vi "Experiment04.vi"() -> ()   [LabVIEW 2009]
uses:
  <vilib>/imath/engines/lvmath2/RunTimeEngine/ErrorHandling/NIMS_Finalize Error.vi
  <vilib>/imath/engines/lvmath2/RunTimeEngine/Parser/MC_Version.vi
  <vilib>/imath/engines/lvmath2/RunTimeEngine/Managers/WorkSpace/UID Generator.vi
  <vilib>/imath/engines/lvmath2/RunTimeEngine/NodeEndStatement/NIMS_NodeEndStatement_Output.vi
  <instcachedir>/0/NIMS_NodeEndStatement_Output_B70DDD75627E4997AAE11E9955EDAA25.lvgen/NIMS_NodeEndStatement_Output_B70DDD75627E4997AAE11E9955EDAA25_000.vi
  <vilib>/imath/engines/lvmath2/RunTimeEngine/Managers/SymbolTable/Clear UID.vi
  <vilib>/imath/engines/lvmath2/RunTimeEngine/LocalVariableDefStatement/MC_LocalVariableDefStatement_Display.vi
  <vilib>/imath/engines/lvmath2/RunTimeEngine/RunTimeType/NIMS_RunTimeType_From StrictType (excl LVString).vi
  <vilib>/imath/engines/lvmath2/RunTimeEngine/RangeToken/NIMS_Range.vi
  <instcachedir>/0/NIMS_Range_6D647EC16A744C98B5DE1D649A2D648D.lvgen/NIMS_Range_6D647EC16A744C98B5DE1D649A2D648D_001.vi
  <vilib>/imath/engines/lvmath/Functions/Error Handling/error.ctl
  <vilib>/imath/engines/lvmath/Functions/Error Handling/MergeErrorsWrapper.vi
  <vilib>/imath/engines/lvmath2/RunTimeEngine/VariableToken/NIMS_VariableToken_CondDefined.vi
  <instcachedir>/0/NIMS_VariableToken_CondDefined_5641E79000FB4D628475532441475385.lvgen/NIMS_VariableToken_CondDefined_5641E79000FB4D628475532441475385_001.vi
  <vilib>/imath/engines/lvmath/Functions/Error Handling/MC_Mask_Errors.vi
  <vilib>/imath/engines/lvmath2/RunTimeEngine/BuiltInFunctions/rem/NIMS_rem_no checks.vi
  <instcachedir>/0/NIMS_rem_no checks_4CC9B305AB7E42EF90AFC4973FB32F8D.lvgen/NIMS_rem_no checks_4CC9B305AB7E42EF90AFC4973FB32F8D_000.vi
  <vilib>/imath/engines/lvmath2/RunTimeEngine/BuiltInFunctions/uint32/NIMS_uint32(real).vi
  <instcachedir>/0/NIMS_uint32(real)_FDC83D68D45943DDB8F3F934FF8A712F.lvgen/NIMS_uint32(real)_FDC83D68D45943DDB8F3F934FF8A712F_000.vi
  <vilib>/imath/engines/lvmath2/RunTimeEngine/BuiltInFunctions/double/NIMS_double.vi
  <instcachedir>/0/NIMS_double_2CE444F3CE4146B199A482FE12545E45.lvgen/NIMS_double_2CE444F3CE4146B199A482FE12545E45_000.vi
  <vilib>/imath/engines/lvmath2/RunTimeEngine/BuiltInFunctions/length/NIMS_length(GV).vi
  <instcachedir>/0/NIMS_length(GV)_7D6E94E728E145E68721C53861296D96.lvgen/NIMS_length(GV)_7D6E94E728E145E68721C53861296D96_000.vi
  <instcachedir>/0/NIMS_Range_6D647EC16A744C98B5DE1D649A2D648D.lvgen/NIMS_Range_6D647EC16A744C98B5DE1D649A2D648D_000.vi
  <vilib>/imathl/engines/lvmath/Functions/Error Handling/Create Error.vi
  <vilib>/imath/engines/lvmath2/RunTimeEngine/ReplaceToken/NIMS_Replace - V(S)=S.vi
  <instcachedir>/0/NIMS_Replace - V(S)=S_670A9E0533664C1D848C8E58B3321B6A.lvgen/NIMS_Replace - V(S)=S_670A9E0533664C1D848C8E58B3321B6A_002.vi
  <vilib>/imath/engines/lvmath2/RunTimeEngine/ReplaceToken/NIMS_Replace - Size Check _(_)=S.vi
  <instcachedir>/0/NIMS_Replace - Size Check _(_)=S_8596181D73404097BAB9CBB006194BB0.lvgen/NIMS_Replace - Size Check _(_)=S_8596181D73404097BAB9CBB006194BB0_002.vi
  <vilib>/imath/engines/lvmath2/RunTimeEngine/ReplaceToken/NIMS_Replace - Check Linear.vi
  <instcachedir>/0/NIMS_Replace - Check Linear_9243CBB174894FF6977027453DA6955E.lvgen/NIMS_Replace - Check Linear_9243CBB174894FF6977027453DA6955E_002.vi
  <vilib>/imath/engines/lvmath2/RunTimeEngine/VariableToken/NIMS_VariableToken_CondDefinedDefinedByReplace.vi
  <instcachedir>/0/NIMS_VariableToken_CondDefinedDefinedByReplace_D162CFFC24174562A9FEA619A91E1A56.lvgen/NIMS_VariableToken_CondDefinedDefinedByReplace_D162CFFC24174562A9FEA619A91E1A56_002.vi
  <vilib>/imath/engines/lvmath2/RunTimeEngine/CommandStatement/MC_CommandStatement_break.vi
  <vilib>/imath/engines/lvmath2/RunTimeEngine/ArithmeticOperatorToken/NIMS_ArithmeticOperator_times.vi
  <instcachedir>/0/NIMS_ArithmeticOperator_times_3987BC660D7947CD8628C10658A43225.lvgen/NIMS_ArithmeticOperator_times_3987BC660D7947CD8628C10658A43225_001.vi
  <instcachedir>/0/NIMS_NodeEndStatement_Output_B70DDD75627E4997AAE11E9955EDAA25.lvgen/NIMS_NodeEndStatement_Output_B70DDD75627E4997AAE11E9955EDAA25_001.vi
  <instcachedir>/0/NIMS_ArithmeticOperator_times_3987BC660D7947CD8628C10658A43225.lvgen/NIMS_ArithmeticOperator_times_3987BC660D7947CD8628C10658A43225_000.vi
  <vilib>/imath/engines/lvmath2/RunTimeEngine/VariableToken/Read/NIMS_Get Elements - RV(_) - Check.vi
  <instcachedir>/0/NIMS_Get Elements - RV(_) - Check_60F12861D0564803969A5D0D0D1716CD.lvgen/NIMS_Get Elements - RV(_) - Check_60F12861D0564803969A5D0D0D1716CD_000.vi
  <instcachedir>/0/NIMS_VariableToken_CondDefined_5641E79000FB4D628475532441475385.lvgen/NIMS_VariableToken_CondDefined_5641E79000FB4D628475532441475385_000.vi
  <instcachedir>/0/NIMS_VariableToken_CondDefined_5641E79000FB4D628475532441475385.lvgen/NIMS_VariableToken_CondDefined_5641E79000FB4D628475532441475385_003.vi
  <vilib>/imath/engines/lvmath2/RunTimeEngine/ArithmeticOperatorToken/NIMS_ArithmeticOperator_power(S).vi
  <instcachedir>/0/NIMS_ArithmeticOperator_power(S)_A502679C095F4520BDC53E297C98A9BD.lvgen/NIMS_ArithmeticOperator_power(S)_A502679C095F4520BDC53E297C98A9BD_000.vi
  <vilib>/imath/engines/lvmath2/RunTimeEngine/BuiltInFunctions/abs/NIMS_abs(signed).vi
  <instcachedir>/0/NIMS_abs(signed)_C4FCB8E6058B49B797C7C8D53CA5F6EC.lvgen/NIMS_abs(signed)_C4FCB8E6058B49B797C7C8D53CA5F6EC_000.vi
  <instcachedir>/0/NIMS_Replace - V(S)=S_670A9E0533664C1D848C8E58B3321B6A.lvgen/NIMS_Replace - V(S)=S_670A9E0533664C1D848C8E58B3321B6A_001.vi
  <instcachedir>/0/NIMS_Replace - Size Check _(_)=S_8596181D73404097BAB9CBB006194BB0.lvgen/NIMS_Replace - Size Check _(_)=S_8596181D73404097BAB9CBB006194BB0_001.vi
  <instcachedir>/0/NIMS_Replace - Check Linear_9243CBB174894FF6977027453DA6955E.lvgen/NIMS_Replace - Check Linear_9243CBB174894FF6977027453DA6955E_001.vi
  <instcachedir>/0/NIMS_VariableToken_CondDefinedDefinedByReplace_D162CFFC24174562A9FEA619A91E1A56.lvgen/NIMS_VariableToken_CondDefinedDefinedByReplace_D162CFFC24174562A9FEA619A91E1A56_001.vi
  <instcachedir>/0/NIMS_Replace - V(S)=S_670A9E0533664C1D848C8E58B3321B6A.lvgen/NIMS_Replace - V(S)=S_670A9E0533664C1D848C8E58B3321B6A_000.vi
  <instcachedir>/0/NIMS_Replace - Size Check _(_)=S_8596181D73404097BAB9CBB006194BB0.lvgen/NIMS_Replace - Size Check _(_)=S_8596181D73404097BAB9CBB006194BB0_000.vi
  <instcachedir>/0/NIMS_Replace - Check Linear_9243CBB174894FF6977027453DA6955E.lvgen/NIMS_Replace - Check Linear_9243CBB174894FF6977027453DA6955E_000.vi
  <instcachedir>/0/NIMS_VariableToken_CondDefinedDefinedByReplace_D162CFFC24174562A9FEA619A91E1A56.lvgen/NIMS_VariableToken_CondDefinedDefinedByReplace_D162CFFC24174562A9FEA619A91E1A56_000.vi
  <instcachedir>/0/NIMS_abs(signed)_C4FCB8E6058B49B797C7C8D53CA5F6EC.lvgen/NIMS_abs(signed)_C4FCB8E6058B49B797C7C8D53CA5F6EC_001.vi
  <instcachedir>/0/NIMS_NodeEndStatement_Output_B70DDD75627E4997AAE11E9955EDAA25.lvgen/NIMS_NodeEndStatement_Output_B70DDD75627E4997AAE11E9955EDAA25_002.vi
  <vilib>/imath/engines/lvmath2/RunTimeEngine/Managers/SymbolTable/NIMS_WorkSpace.lvlib
panel:
  out "Current VI path 10":string
  out "New Path for Picture 10":string
  out "Part Stripped 10":string
  out "Stripped Path 10":string
  out "Current VI path 9":string
  out "New Path for Picture 9":string
  out "Part Stripped 9":string
  out "Stripped Path 9":string
  out "Current VI path 8":string
  out "New Path for Picture 8":string
  out "Part Stripped 8":string
  out "Stripped Path 8":string
  out "Current VI path 7":string
  out "New Path for Picture 7":string
  out "Part Stripped 7":string
  out "Stripped Path 7":string
  out "Current VI path 6":string
  out "New Path for Picture 6":string
  out "Part Stripped 6":string
  out "Stripped Path 6":string
  out "Current VI path 5":string
  out "New Path for Picture 5":string
  out "Part Stripped 5":string
  out "Stripped Path 5":string
  out "Current VI path 4":string
  out "New Path for Picture 4":string
  out "Part Stripped 4":string
  out "Stripped Path 4":string
  out "Current VI path 3":string
  out "New Path for Picture 3":string
  out "Part Stripped 3":string
  out "Stripped Path 3":string
  out "Current VI path 2":string
  out "New Path for Picture 2":string
  out "Part Stripped 2":string
  out "Stripped Path 2":string
  out "Current VI path":string
  out "New Path for Picture":string
  out "Part Stripped":string
  out "Stripped Path":string
  out "error out":errorcluster
  out "error out":errorcluster
  out "error out":errorcluster
  out "error out":errorcluster
  in  "?":enum32{"CAVITY"}(tab)
  in  "FIRST 3dB POINT":bool
  in  "?":dbl(slide) scale=8.0..12.5 scale format="%#.6g"
  out "Qdesigned":dbl
  in  "RESONANT FREQUENCY":dbl(slide) scale=8.5..12.0
  out "?":errorcluster
  out "XY Graph":cluster{"Y":dbl[], "Y":dbl[]}[](graph)
  out "frequency":dbl
  out "power(dB)":cdb
  in  "SECOND 3dB POINT":bool
  in  "BAND WIDTH":bool
  in  "Q FACTOR":bool
  in  "POWER(dB) at RESONANCE":bool
  out "?":dbl
  out "?":dbl
  out "?":dbl
  out "?":dbl
  out "?":dbl
  in  "HELP FOR CAVITY":bool
  in  "?":enum32{"ATTENUATOR"}(tab)
  out "?":dbl[](graph)
  in  "Set the value of attenuation in dB":dbl(slide) scale=0.0..100.0
  out "?":errorcluster
  in  "HELP FOR ATTENUATOR":bool
  out "error out":errorcluster
  in  "?":enum32{"ISOLATOR"}(tab)
  out "?":dbl[](graph)
  in  "?":bool
  out "?":errorcluster
  in  "HELP FOR ISOLATOR":bool
  in  "?":enum32{"MODULATOR"}(tab)
  out "?":dbl[](graph)
  in  "Modulating Frequency(KHz)":dbl(slide) scale=0.5..1.5
  out "?":errorcluster
  in  "HELP FOR MODULATOR":bool
  in  "?":enum32{"SOURCE"}(tab)
  out "?":dbl[](graph)
  in  "Frequency of carrier wave(GHz)":dbl(slide) scale=8.2..12.4
  in  "Voltage 3":dbl(knob) scale=0.0..20.0 scale format="%#_10g"
  out "?":errorcluster
  in  "HELP FOR SOURCE":bool
  # "Backward Direction"
  # "Forward direction"
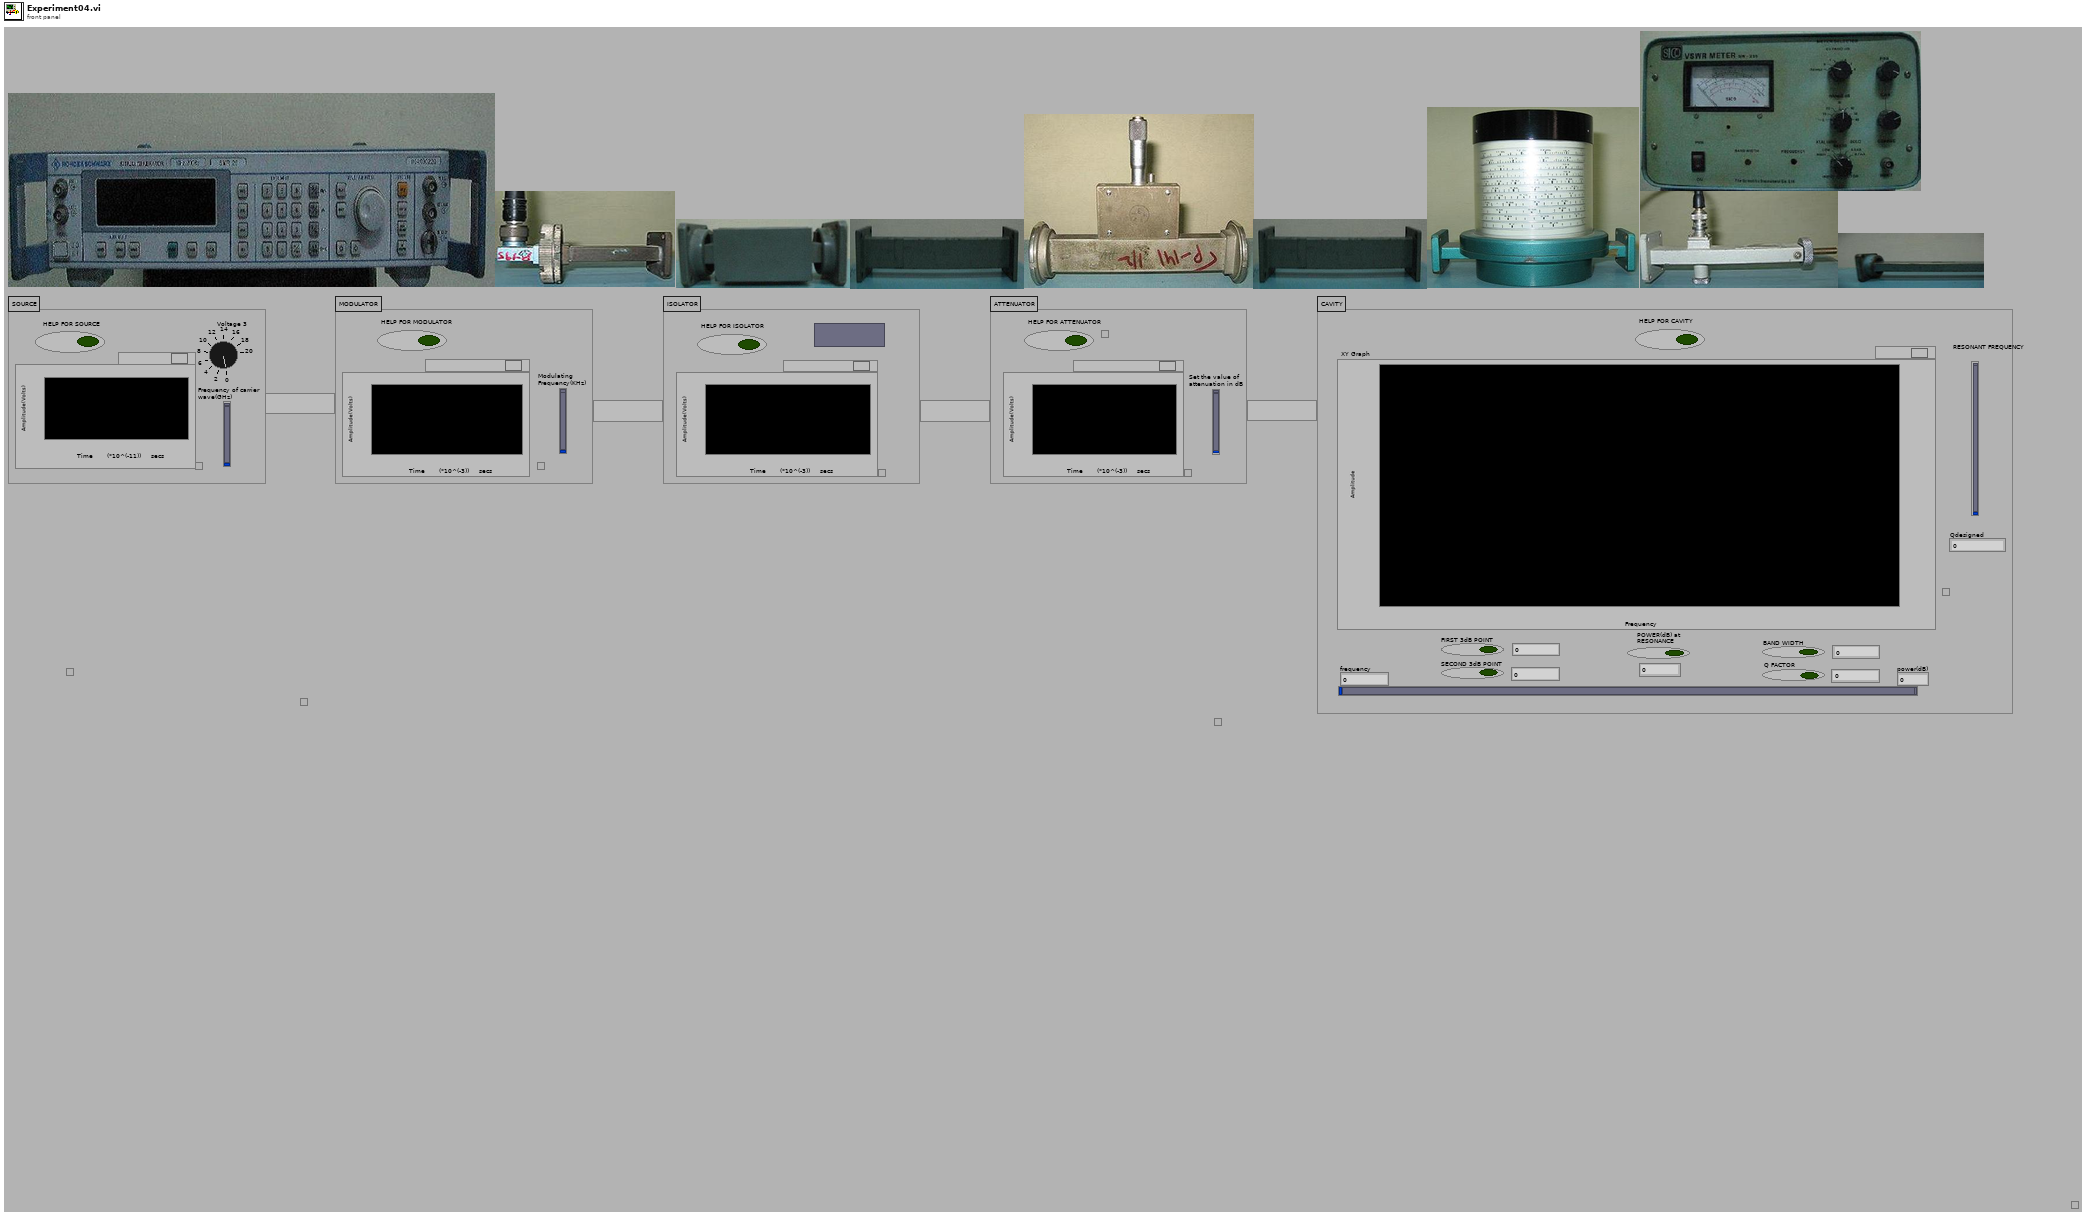
[diagram p1: front panel]
types:
  T1 = typedef "imagedata.ctl" = cluster{"image type":i32, "image depth":i32, "image":u8[], "mask":u8[], "colors":u32[], "Rectangle":cluster{"left":i16, "top":i16, "right":i16, "bottom":i16}}
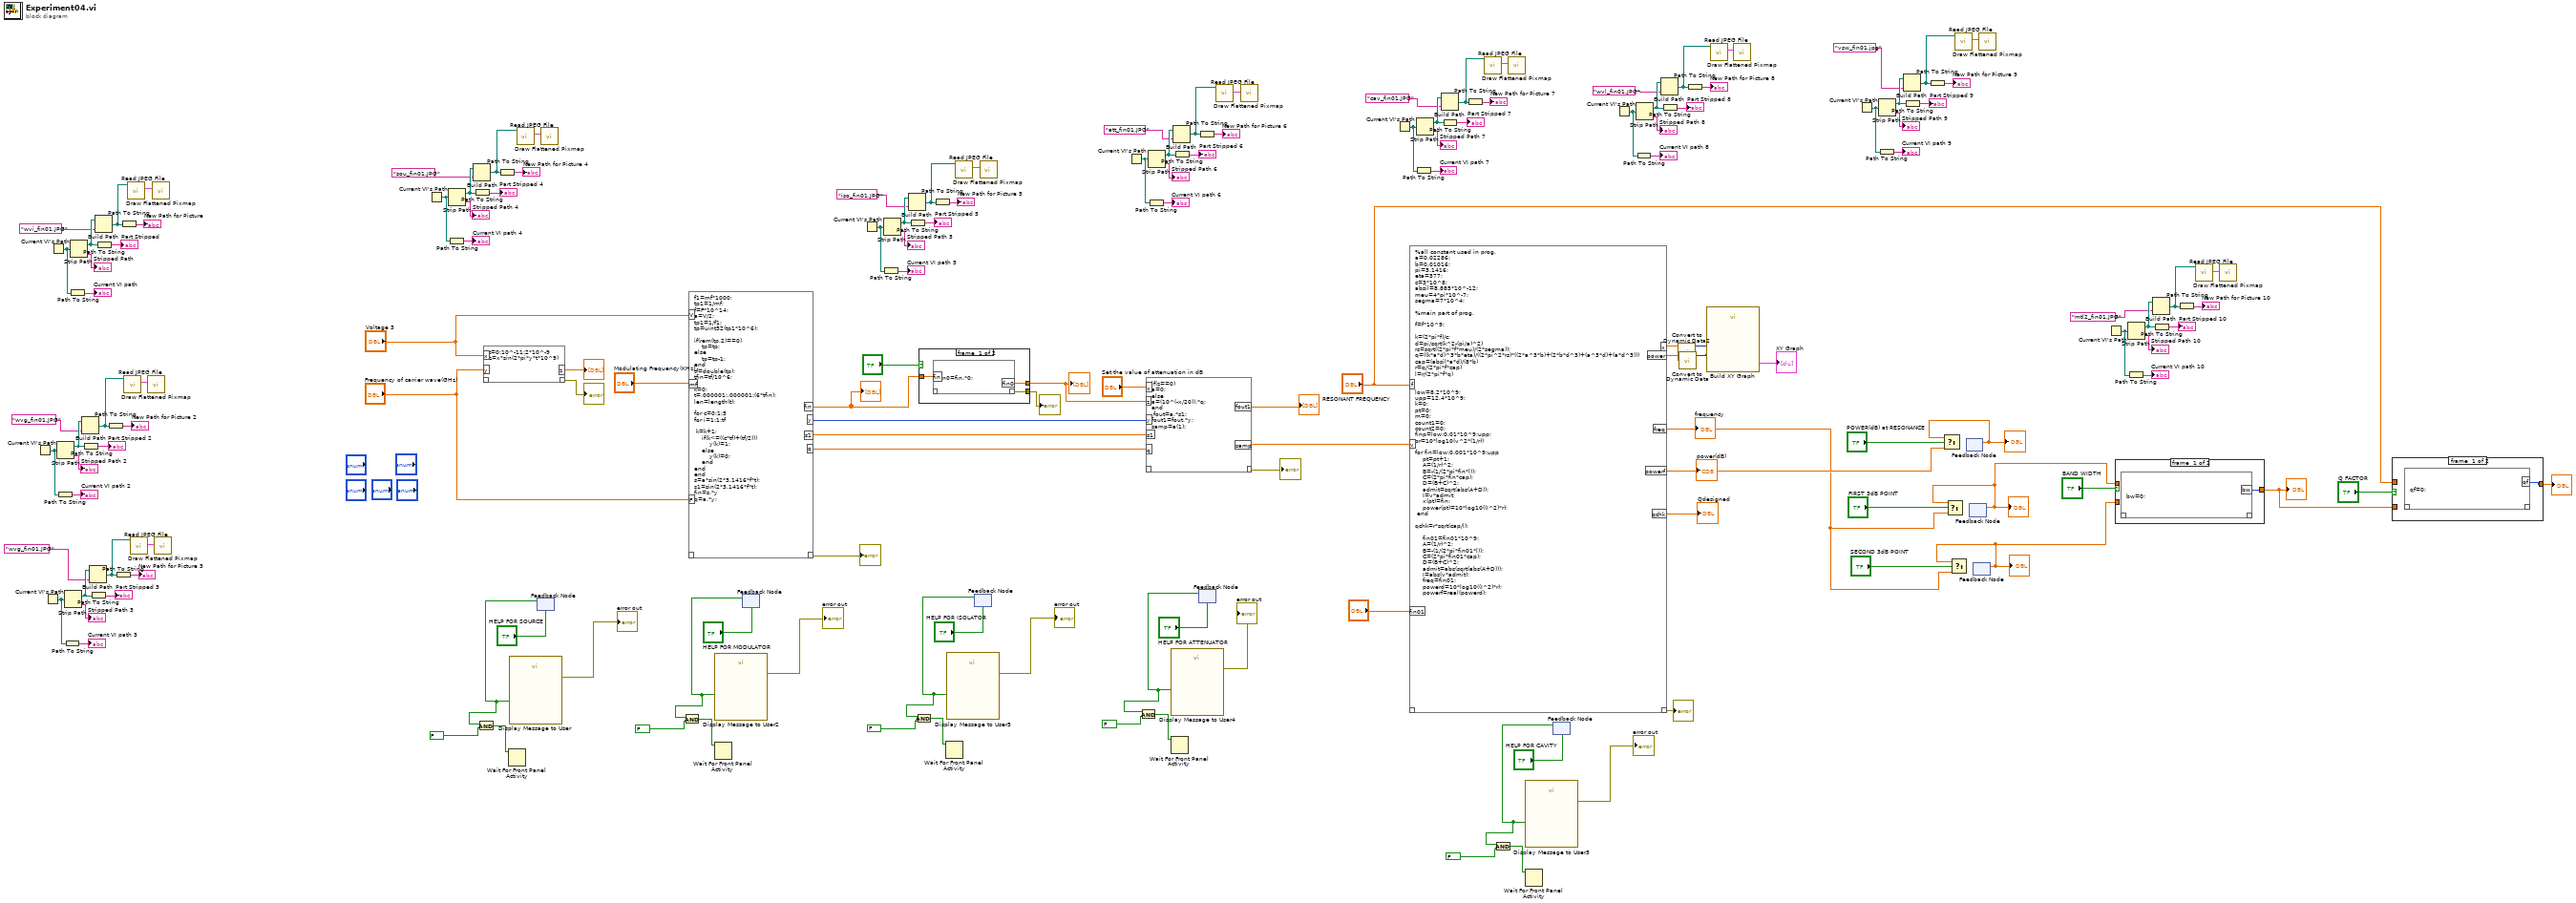
[diagram p0: block diagram]
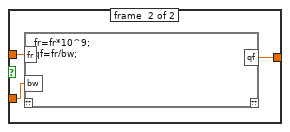
[diagram p2: hidden frame]
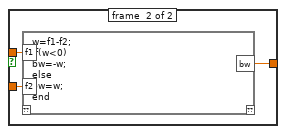
[diagram p3: hidden frame]
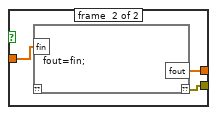
[diagram p4: hidden frame]
diagram:
  n1 = Current VI's Path() -> (path=w67:path)
  n2 = Current VI's Path() -> (path=w59:path)
  n3 = Current VI's Path() -> (path=w75:path)
  n4 = Path To String(path=w67) -> (string=→"Current VI path 2":string)
  n5 = Strip Path(path=w67) -> (stripped path=w72:path, name=→"Stripped Path 2":string)
  n6 = Path To String(path=w59) -> (string=→"Current VI path 3":string)
  n7 = Strip Path(path=w59) -> (stripped path=w64:path, name=→"Stripped Path 3":string)
  n8 = Path To String(path=w75) -> (string=→"Current VI path":string)
  n9 = Strip Path(path=w75) -> (stripped path=w80:path, name=→"Stripped Path":string)
  n10 = Build Path(base path=w72, name or relative path="wvg_fin01.JPG") -> (appended path=w65:path)
  n11 = Path To String(path=w72) -> (string=→"Part Stripped 2":string)
  n12 = Build Path(base path=w64, name or relative path="wvg_fin01.JPG") -> (appended path=w57:path)
  n13 = Path To String(path=w64) -> (string=→"Part Stripped 3":string)
  n14 = Build Path(base path=w80, name or relative path="wvi_fin01.JPG") -> (appended path=w73:path)
  n15 = Path To String(path=w80) -> (string=→"Part Stripped":string)
  n16 = Path To String(path=w65) -> (string=→"New Path for Picture 2":string)
  n17 = Path To String(path=w57) -> (string=→"New Path for Picture 3":string)
  n18 = Path To String(path=w73) -> (string=→"New Path for Picture":string)
  n19 = call <vilib>:"Read JPEG File.vi"("path to JPEG file"=w65) -> ("image data"=w92:T1)  [unwired: 1 in, 9 out]
  n20 = call <vilib>:"Read JPEG File.vi"("path to JPEG file"=w73) -> ("image data"=w95:T1)  [unwired: 1 in, 9 out]
  n21 = call <vilib>:"Read JPEG File.vi"("path to JPEG file"=w57) -> ("image data"=w91:T1)  [unwired: 1 in, 9 out]
  n22 = call <vilib>:"Draw Flattened Pixmap.vi"("image data"=w92) -> ()  [unwired: 1 in, 8 out]
  n23 = call <vilib>:"Draw Flattened Pixmap.vi"("image data"=w95) -> ()  [unwired: 1 in, 8 out]
  n24 = call <vilib>:"Draw Flattened Pixmap.vi"("image data"=w91) -> ()  [unwired: 1 in, 8 out]
  n25 = Current VI's Path() -> (path=w51:path)
  n26 = Path To String(path=w51) -> (string=→"Current VI path 4":string)
  n27 = Strip Path(path=w51) -> (stripped path=w56:path, name=→"Stripped Path 4":string)
  n28 = Build Path(base path=w56, name or relative path="sou_fin01.JPG") -> (appended path=w49:path)
  n29 = Path To String(path=w56) -> (string=→"Part Stripped 4":string)
  n30 = mathscript code="t=0:10^-11:2*10^-9\nz=x*sin(2*pi*y*t*10^9)"("x"="Voltage 3", "y"="Frequency of carrier wave(GHz)") -> ("??"=→"?":errorcluster, "z"=→"?":dbl[])  [unwired: 1 in]
  n31 = Path To String(path=w49) -> (string=→"New Path for Picture 4":string)
  n32 = call <vilib>:"Read JPEG File.vi"("path to JPEG file"=w49) -> ("image data"=w96:T1)  [unwired: 1 in, 9 out]
  n33 = feedback #1("HELP FOR SOURCE") -> (w117:bool)
  n34 = And(x=w117, y=FALSE) -> (x .and. y?=w115:bool)
  n35 = Wait For Front Panel Activity(3:w115) -> ()  [unwired: 3 out]
  n36 = call "Display Message to User"("Enable"=w117) -> ("error out"=→"error out":errorcluster, "CLOSE"=w119:bool)  [unwired: 2 in, 7 out]
  n37 = call <vilib>:"Draw Flattened Pixmap.vi"("image data"=w96) -> ()  [unwired: 1 in, 8 out]
  n38 = mathscript code="f1=mf*1000;\ntp1=1/mf;\nf=F*10^14;\na=V/2;\ntp1=1/f1;\ntp=uint32(tp1*10^6);\n\nif(rem(tp,2)==0)\n    tp=tp;\nelse\n    tp=tp-1;\nend\ntf=double(tp);\ntfin=tf/10^6;\n\nk=0;\nt=.000001:.000001:(6*tfin);\nlen=length(t);\n\nfor c=0:1:5\nfor i=1:1:tf\n  \n k=k+1;\n    if(k<=((c*tf)+(tf/2)))\n        y(k)=1;\n    else\n        y(k)=0;\n    end\nend\nend\ns=a*sin(2*3.1416*f*t);\ns1=sin(2*3.1416*f*t);\nfin=s.*y\nq=a.*y;"("V"="Voltage 3", "mf"="Modulating Frequency(KHz)", "F"="Frequency of carrier wave(GHz)") -> ("??"=→"?":errorcluster, "y"=w147:i32[], "q"=w145:dbl[], "fin"=w152:dbl[], "s1"=w146:dbl[])  [unwired: 1 in]
  "?" <- w152
  n39 = feedback #2("HELP FOR MODULATOR") -> (w111:bool)
  n40 = And(x=w111, y=FALSE) -> (x .and. y?=w109:bool)
  n41 = Wait For Front Panel Activity(3:w109) -> ()  [unwired: 3 out]
  n42 = call "Display Message to User2"("Enable"=w111) -> ("error out"=→"error out":errorcluster, "CLOSE"=w113:bool)  [unwired: 2 in, 7 out]
  n43 = Current VI's Path() -> (path=w43:path)
  n44 = Path To String(path=w43) -> (string=→"Current VI path 5":string)
  n45 = Strip Path(path=w43) -> (stripped path=w48:path, name=→"Stripped Path 5":string)
  n46 = Build Path(base path=w48, name or relative path="iso_fin01.JPG") -> (appended path=w41:path)
  n47 = Path To String(path=w48) -> (string=→"Part Stripped 5":string)
  n48 = case shown="False" "?" {
    tunnel: [w163 w184] -> w148
    tunnel: w152 -> [w164 w185]
    tunnel: [w162 w183] -> w150
    frame #0 {
      n49 = mathscript code="fin0=fin.*0;"("fin"=w164) -> ("??"=w162:errorcluster, "fin0"=w163:dbl[])  [unwired: 1 in]
    }
    frame #1 {
      n50 = mathscript code="fout=fin;"("fin"=w185) -> ("??"=w183:errorcluster, "fout"=w184:dbl[])  [unwired: 1 in]
    }
  }
  "?" <- w148
  "?" <- w150
  n51 = Path To String(path=w41) -> (string=→"New Path for Picture 5":string)
  n52 = call <vilib>:"Read JPEG File.vi"("path to JPEG file"=w41) -> ("image data"=w94:T1)  [unwired: 1 in, 9 out]
  n53 = feedback #3("HELP FOR ISOLATOR") -> (w105:bool)
  n54 = And(x=w105, y=FALSE) -> (x .and. y?=w103:bool)
  n55 = Wait For Front Panel Activity(3:w103) -> ()  [unwired: 3 out]
  n56 = call "Display Message to User3"("Enable"=w105) -> ("error out"=→"error out":errorcluster, "CLOSE"=w107:bool)  [unwired: 2 in, 7 out]
  n57 = call <vilib>:"Draw Flattened Pixmap.vi"("image data"=w94) -> ()  [unwired: 1 in, 8 out]
  n58 = Current VI's Path() -> (path=w35:path)
  n59 = mathscript code="if(z==0)\na=0; \nelse\na=(10^(-x/20)).*q;\nend\n fout=a.*s1;\nfout1=fout.*y;\nsamp=a(1);"("x"="Set the value of attenuation in dB", "z"=w148, "y"=w147, "s1"=w146, "q"=w145) -> ("??"=→"?":errorcluster, "fout1"=→"?":dbl[], "samp"=w157:dbl)  [unwired: 1 in]
  n60 = Path To String(path=w35) -> (string=→"Current VI path 6":string)
  n61 = Strip Path(path=w35) -> (stripped path=w40:path, name=→"Stripped Path 6":string)
  n62 = Build Path(base path=w40, name or relative path="att_fin01.JPG") -> (appended path=w33:path)
  n63 = Path To String(path=w40) -> (string=→"Part Stripped 6":string)
  n64 = Path To String(path=w33) -> (string=→"New Path for Picture 6":string)
  n65 = feedback #4("HELP FOR ATTENUATOR") -> (w99:bool)
  n66 = And(x=w99, y=FALSE) -> (x .and. y?=w97:bool)
  n67 = Wait For Front Panel Activity(3:w97) -> ()  [unwired: 3 out]
  n68 = call "Display Message to User4"("Enable"=w99) -> ("error out"=→"error out":errorcluster, "CLOSE"=w101:bool)  [unwired: 2 in, 7 out]
  n69 = call <vilib>:"Read JPEG File.vi"("path to JPEG file"=w33) -> ("image data"=w93:T1)  [unwired: 1 in, 9 out]
  n70 = call <vilib>:"Draw Flattened Pixmap.vi"("image data"=w93) -> ()  [unwired: 1 in, 8 out]
  n71 = Current VI's Path() -> (path=w27:path)
  n72 = mathscript code="%all constant used in prog.\na=0.02286;\nb=0.01016;\npi=3.1416;\neta=377;\nc=3*10^8;\nabsil=8.885*10^-12;\nmeu=4*pi*10^-7;\nsegma=7*10^4;\n\n%main part of prog.\n\nf=f*10^9;\n\nk=(2*pi*f)/c;\nd=pi/sqrt(k^2-(pi/a)^2)\nrs=sqrt((2*pi*f*meu)/(2*segma));\nq=((k*a*d)^3*b*eta)/((2*pi^2*rs)*((2*a^3*b)+(2*b*d^3)+(a^3*d)+(a*d^3)))\ncap=(absil*a*d)/(8*b)\nr=q/(2*pi*f*cap)\nl=r/(2*pi*f*q)\n\n\nlow=8.2*10^9;\nupp=12.4*10^9;\nk=0;\npt=0;\nm=0;\ncount1=0;\ncount2=0;\nfinp=low:0.01*10^9:upp;\npr=10*log10(v^2*(1/r))\n\nfor fin=low:0.001*10^9:upp\n    pt=pt+1;\n    A=(1/r)^2;\n    B=-(1/(2*pi*fin*l));\n    C=(2*pi*fin*cap);\n    D=(B+C)^2;\n    admit=sqrt(abs(A+D));\n    I=v*admit;\n    x(pt)=fin;\n    power(pt)=10*log10((I^2)*r);\n end\n\nqchk=r*sqrt(cap/l);\n    \n    fin01=fin01*10^9;\n    A=(1/r)^2;\n    B=-(1/(2*pi*fin01*l));\n    C=(2*pi*fin01*cap);\n    D=(B+C)^2;\n    admit=abs(sqrt(abs(A+D)));\n    I=abs(v*admit);\n    freq=fin01;\n    powerd=10*log10((I^2)*r);\n    powerf=real(powerd);"("v"=w157, "f"="RESONANT FREQUENCY", "fin01"="?") -> ("??"=→"?":errorcluster, "power"=w141:dbl[], "qchk"=→"Qdesigned":dbl, "x"=w139:dbl[], "freq"=w129:dbl, "powerf"=w134:dbl)  [unwired: 1 out]
  "frequency" <- w129
  "power(dB)" <- w134
  n73 = Path To String(path=w27) -> (string=→"Current VI path 7":string)
  n74 = Strip Path(path=w27) -> (stripped path=w32:path, name=→"Stripped Path 7":string)
  n75 = Build Path(base path=w32, name or relative path="cav_fin01.JPG") -> (appended path=w25:path)
  n76 = Path To String(path=w32) -> (string=→"Part Stripped 7":string)
  n77 = Path To String(path=w25) -> (string=→"New Path for Picture 7":string)
  n78 = call <vilib>:"Read JPEG File.vi"("path to JPEG file"=w25) -> ("image data"=w84:T1)  [unwired: 1 in, 9 out]
  n79 = call <vilib>:"Draw Flattened Pixmap.vi"("image data"=w84) -> ()  [unwired: 1 in, 8 out]
  n80 = feedback #5("HELP FOR CAVITY") -> (w87:bool)
  n81 = And(x=w87, y=FALSE) -> (x .and. y?=w85:bool)
  n82 = Wait For Front Panel Activity(3:w85) -> ()  [unwired: 3 out]
  n83 = call "Display Message to User5"("Enable"=w87) -> ("error out"=→"error out":errorcluster, "CLOSE"=w89:bool)  [unwired: 2 in, 7 out]
  n84 = Current VI's Path() -> (path=w19:path)
  n85 = Path To String(path=w19) -> (string=→"Current VI path 8":string)
  n86 = Strip Path(path=w19) -> (stripped path=w24:path, name=→"Stripped Path 8":string)
  n87 = Build Path(base path=w24, name or relative path="wvl_fin01.JPG") -> (appended path=w17:path)
  n88 = Path To String(path=w24) -> (string=→"Part Stripped 8":string)
  n89 = call "Convert to Dynamic Data2"("Array"=w139) -> ("Dynamic Data Type"=w138:dynamicdata)  [unwired: 3 in]
  n90 = call "Convert to Dynamic Data"("Array"=w141) -> ("Dynamic Data Type"=w140:dynamicdata)  [unwired: 3 in]
  n91 = Path To String(path=w17) -> (string=→"New Path for Picture 8":string)
  n92 = call "Build XY Graph"("Y Input"=w140, "X Input"=w138) -> ("XY Graph"=→"XY Graph":cluster{"Y":dbl[], "Y":dbl[]}[])  [unwired: 8 in, 1 out]
  n93 = call <vilib>:"Read JPEG File.vi"("path to JPEG file"=w17) -> ("image data"=w83:T1)  [unwired: 1 in, 9 out]
  n94 = call <vilib>:"Draw Flattened Pixmap.vi"("image data"=w83) -> ()  [unwired: 1 in, 8 out]
  n95 = Current VI's Path() -> (path=w11:path)
  n96 = Path To String(path=w11) -> (string=→"Current VI path 9":string)
  n97 = Strip Path(path=w11) -> (stripped path=w16:path, name=→"Stripped Path 9":string)
  n98 = Build Path(base path=w16, name or relative path="vsw_fin01.jpg") -> (appended path=w9:path)
  n99 = Path To String(path=w16) -> (string=→"Part Stripped 9":string)
  n100 = Path To String(path=w9) -> (string=→"New Path for Picture 9":string)
  n101 = call <vilib>:"Read JPEG File.vi"("path to JPEG file"=w9) -> ("image data"=w82:T1)  [unwired: 1 in, 9 out]
  n102 = feedback #6() -> (w127:dbl)  [unwired: 1 in]
  "?" <- w127
  n103 = Select(t=w127, s="POWER(dB) at RESONANCE", f=w134) -> (s? t:f=w136:dbl)
  n104 = feedback #7() -> (w122:dbl)  [unwired: 1 in]
  "?" <- w122
  n105 = Select(t=w122, s="FIRST 3dB POINT", f=w129) -> (s? t:f=w133:dbl)
  n106 = feedback #8() -> (w121:dbl)  [unwired: 1 in]
  "?" <- w121
  n107 = Select(t=w121, s="SECOND 3dB POINT", f=w129) -> (s? t:f=w131:dbl)
  n108 = call <vilib>:"Draw Flattened Pixmap.vi"("image data"=w82) -> ()  [unwired: 1 in, 8 out]
  n109 = Current VI's Path() -> (path=w3:path)
  n110 = case shown="True" "BAND WIDTH" {
    tunnel: w121 -> [_ w219]
    tunnel: [w202 w218] -> w124
    tunnel: w122 -> [_ w217]
    frame #0 {
      n111 = mathscript code="bw=0;"() -> ("bw"=w202:i32)  [unwired: 1 in, 1 out]
    }
    frame #1 {
      n112 = mathscript code="w=f1-f2;\nif(w<0)\nbw=-w;\nelse\nbw=w;\nend"("f1"=w217, "f2"=w219) -> ("bw"=w218:dbl)  [unwired: 1 in, 1 out]
    }
  }
  "?" <- w124
  n113 = Path To String(path=w3) -> (string=→"Current VI path 10":string)
  n114 = Strip Path(path=w3) -> (stripped path=w8:path, name=→"Stripped Path 10":string)
  n115 = Build Path(base path=w8, name or relative path="mtl2_fin01.JPG" ("name or relative path 2")) -> (appended path=w1:path)
  n116 = Path To String(path=w8) -> (string=→"Part Stripped 10":string)
  n117 = Path To String(path=w1) -> (string=→"New Path for Picture 10":string)
  n118 = call <vilib>:"Read JPEG File.vi"("path to JPEG file"=w1) -> ("image data"=w81:T1)  [unwired: 1 in, 9 out]
  n119 = call <vilib>:"Draw Flattened Pixmap.vi"("image data"=w81) -> ()  [unwired: 1 in, 8 out]
  n120 = case shown="True" "Q FACTOR" {
    tunnel: "RESONANT FREQUENCY" -> [_ w277]
    tunnel: w124 -> [_ w276]
    tunnel: [w260 w275] -> w123
    frame #0 {
      n121 = mathscript code="qf=0;"() -> ("qf"=w260:i32)  [unwired: 1 in, 1 out]
    }
    frame #1 {
      n122 = mathscript code="fr=fr*10^9;\nqf=fr/bw;"("fr"=w277, "bw"=w276) -> ("qf"=w275:dbl)  [unwired: 1 in, 1 out]
    }
  }
  "?" <- w123
